vi "OpenMV_SelectLab.vi"(2 "ROI":T1, 3 "image":picture) -> (0 "ROI out":T1, 1 "thresholds":dbl[](array[numeric])=[90.0, 10.0, 20.0, -20.0, 20.0, -20.0])   [LabVIEW 2017]
doc: "This VI pops up a window where the user can select a region of interest."
panel:
  out "Plots":T2
  out "Mouse Down":cluster{"X":i32, "Y":i32}
  out "String":string
  out "Mouse in":bool
  in  "Pen":u32(colorbox)=16774656
  out "overlay":picture caption="Image"
  in  "OK":bool
  out "Display":picture caption="new picture"
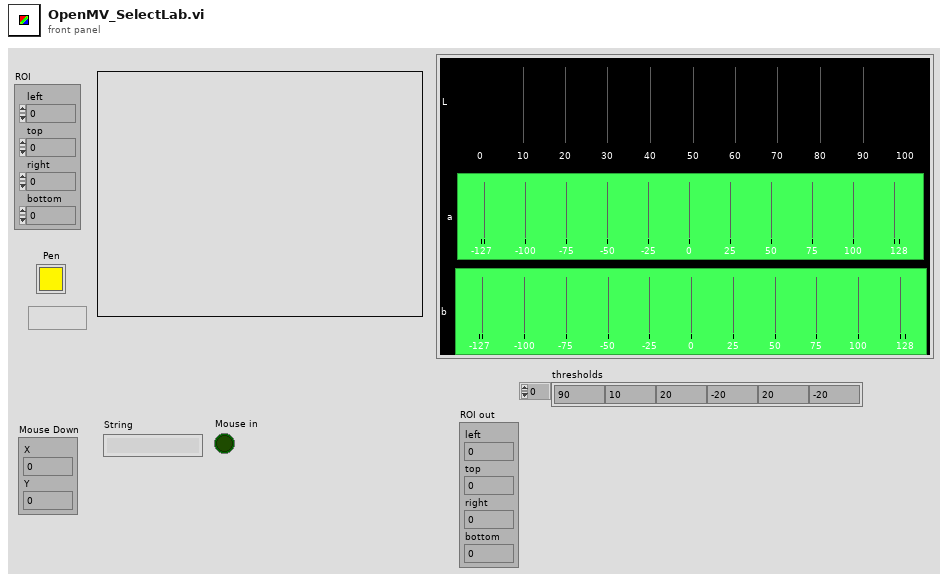
[diagram p1: front panel]
types:
  T1 = cluster{"left":i32, "top":i32, "right":i32, "bottom":i32}
  T2 = cluster{"L":dbl[], "a":cluster{i32, i32, dbl[]}, "b":cluster{i32, i32, dbl[]}}
  T3 = typedef "imagedata.ctl" = cluster{"image type":i32, "image depth":i32, "image":u8[], "mask":u8[], "colors":u32[], "Rectangle":cluster{"left":i16, "top":i16, "right":i16, "bottom":i16}}
  T4 = typedef "LVMouseTypeDef.ctl" = cluster{"Mouse Position":cluster{"X":i32, "Y":i32}, "Mouse Modifiers":cluster{"Button Down":bool, "Shift Mod":bool, "Menu Mod":bool, "Option Mod":bool}}
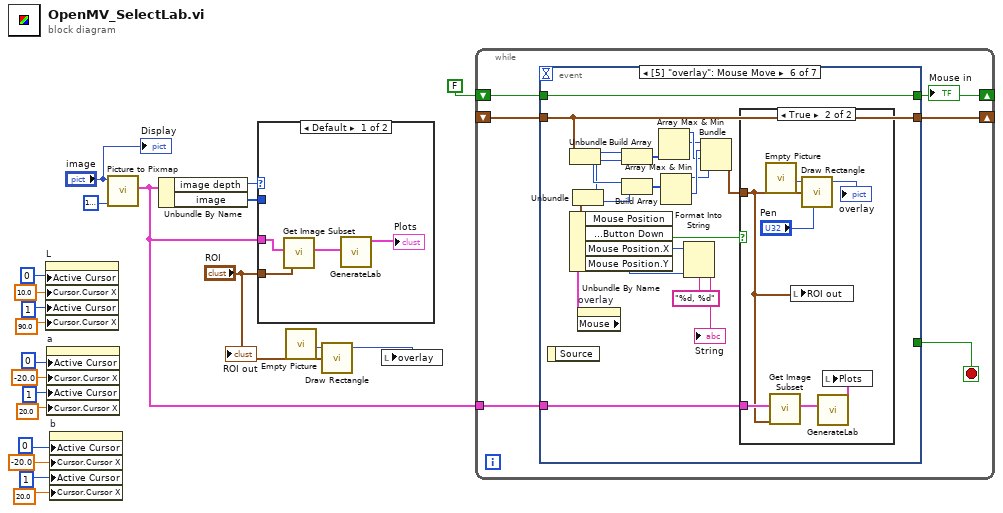
[diagram p0: block diagram]
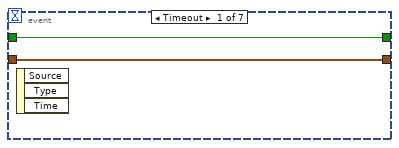
[diagram p3: hidden frame]
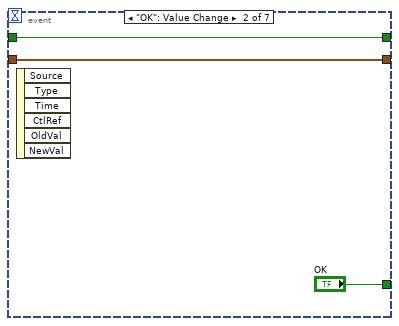
[diagram p4: hidden frame]
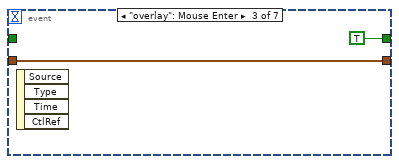
[diagram p5: hidden frame]
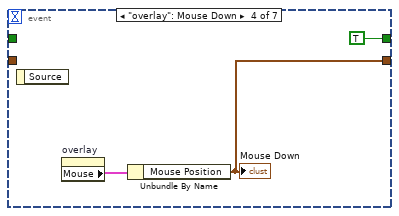
[diagram p6: hidden frame]
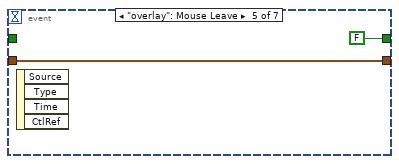
[diagram p7: hidden frame]
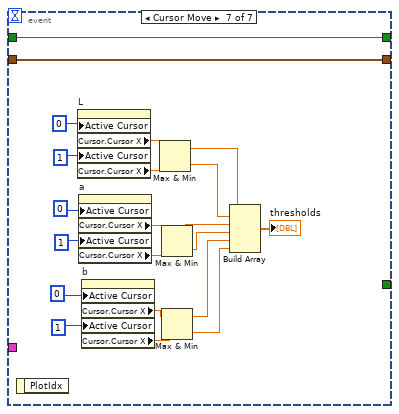
[diagram p9: hidden frame]
diagram:
  n1 = property on="L" class="WFGraph (strict)"("Active Cursor"=u32 0, "Cursor.Cursor X"=10.0 ("Cursor.Cursor Position:Cursor X"), "Active Cursor"=u32 1, "Cursor.Cursor X"=90.0 ("Cursor.Cursor Position:Cursor X")) -> ()  [unwired: 2 in, 2 out]
  n2 = property on="a" class="WFGraph (strict)"("Active Cursor"=u32 0, "Cursor.Cursor X"=-20.0 ("Cursor.Cursor Position:Cursor X"), "Active Cursor"=u32 1, "Cursor.Cursor X"=20.0 ("Cursor.Cursor Position:Cursor X")) -> ()  [unwired: 2 in, 2 out]
  n3 = property on="b" class="WFGraph (strict)"("Active Cursor"=u32 0, "Cursor.Cursor X"=-20.0 ("Cursor.Cursor Position:Cursor X"), "Active Cursor"=u32 1, "Cursor.Cursor X"=20.0 ("Cursor.Cursor Position:Cursor X")) -> ()  [unwired: 2 in, 2 out]
  n4 = call <vilib>:"Picture to Pixmap.vi"("Background Color"=u32 16777216, "picture"="image") -> ("image data"=w16:T3)  [unwired: 8 in, 1 out]
  n5 = Unbundle By Name(w16) -> ("image depth"=w19:i32, "image"=w18:u8[])
  n6 = case shown="Default" w19 {
    tunnel: w18 -> [_ _]
    tunnel: w16 -> [w24 _]
    tunnel: "ROI" -> [w22 _]
    frame Default {
      n7 = call <vilib>:"Get Image Subset.vi"("subset rect"=w22, "image data"=w24) -> ("image subset"=w23:T3)  [unwired: 4 in, 1 out]
      n8 = call "GenerateLab.vi"("image data"=w23) -> ("Plots"=→"Plots":T2)  [unwired: 9 in, 1 out]
    }
    frame ..8 {
    }
  }
  n9 = call "Empty Picture"() -> ("empty picture"=w3:picture)
  n10 = call <vilib>:"Draw Rectangle.vi"("picture"=w3, "rect"="ROI") -> ("new picture"=w1:picture)  [unwired: 7 in]
  n11 = local write "overlay"(w1) -> ()
  n12 = while {
    shift-right: [w30] -> _
    shift-left: FALSE ("Mouse in") -> [w29]
    shift-right: [w28] -> _
    shift-left: _ -> [w27]
    tunnel: w16 -> [w26]
    stop <- w31 stop-if-true
    n13 = event shown="[5] \"overlay\": Mouse Move" {
      selector: _ -> [_ _ _ _ _ _ _]
      dyn-events: _ -> [_ _ _ _ _ _ _]
      timeout: _ -> [_ _ _ _ _ _ _]
      tunnel: [_ "OK" _ _ _ _ _] -> w31
      tunnel: [w33 w35 TRUE ("Mouse in") TRUE ("Mouse in") FALSE ("Mouse in") w64 w91] -> w30
      tunnel: w29 -> [w33 w35 _ _ _ w64 w91]
      tunnel: [w32 w34 w37 w39 w42 w52 w92] -> w28
      tunnel: w27 -> [w32 w34 w37 _ w42 w52 w92]
      tunnel: w26 -> [_ _ _ _ _ w44 _]
      event Timeout {
        n14 = event-data() -> ()  [unwired: 1 in, 3 out]
      }
      event "OK": Value Change {
        n15 = event-data() -> ()  [unwired: 1 in, 6 out]
      }
      event "overlay": Mouse Enter {
        n16 = event-data() -> ()  [unwired: 1 in, 4 out]
      }
      event "overlay": Mouse Down {
        n17 = event-data() -> ()  [unwired: 1 in, 1 out]
        n18 = property on="overlay" class="Pict"() -> ("Mouse"=w40:T4)  [unwired: 2 in, 2 out]
        n19 = Unbundle By Name(w40) -> ("Mouse Position"=w39:cluster{"X":i32, "Y":i32})
        "Mouse Down" <- w39
      }
      event "overlay": Mouse Leave {
        n20 = event-data() -> ()  [unwired: 1 in, 4 out]
      }
      event "overlay": Mouse Move {
        n21 = event-data() -> ()  [unwired: 1 in, 1 out]
        n22 = Unbundle(w52) -> ("X"=w53:i32, "Y"=w51:i32)
        n23 = property on="overlay" class="Pict"() -> ("Mouse"=w63:T4)  [unwired: 2 in, 2 out]
        n24 = Unbundle By Name(w63) -> ("Mouse Position"=w48:cluster{"X":i32, "Y":i32}, "Mouse Modifiers.Button Down"=w62:bool, "Mouse Position.X"=w60:i32, "Mouse Position.Y"=w59:i32)
        n25 = Unbundle(w48) -> ("X"=w47:i32, "Y"=w46:i32)
        n26 = Build Array(w53, w47) -> (w50:i32[])
        n27 = Build Array(w51, w46) -> (w49:i32[])
        n28 = Array Max & Min(array=w50) -> (max value=w55:i32, min value=w54:i32)  [unwired: 2 out]
        n29 = Array Max & Min(array=w49) -> (max value=w56:i32, min value=w57:i32)  [unwired: 2 out]
        n30 = Format Into String(format string="%d, %d", w60, w59) -> (resulting string=→"String":string)  [unwired: 2 in, 1 out]
        n31 = Bundle(w54, w57, w55, w56) -> (w45:cluster{i32, i32, i32, i32})  [unwired: 1 out]
        n32 = case shown="True" w62 {
          tunnel: w45 -> [_ w65]
          tunnel: w44 -> [_ w68]
          frame False {
          }
          frame True {
            n33 = call "Empty Picture"() -> ("empty picture"=w71:picture)
            n34 = call <vilib>:"Get Image Subset.vi"("subset rect"=w65, "image data"=w68) -> ("image subset"=w67:T3)  [unwired: 4 in, 1 out]
            n35 = local write "ROI out"(w65) -> ()
            n36 = call <vilib>:"Draw Rectangle.vi"("picture"=w71, "rect"=w65, "color(black)"="Pen") -> ("new picture"=→"overlay":picture)  [unwired: 6 in]
            n37 = call "GenerateLab.vi"("image data"=w67) -> ("Plots"=w66:T2)  [unwired: 9 in, 1 out]
            n38 = local write "Plots"(w66) -> ()
          }
        }
      }
      event "Plots.L", "Plots.a", "Plots.b": Cursor Move {
        n39 = event-data() -> ()  [unwired: 1 in, 1 out]
        n40 = property on="L" class="WFGraph (strict)"("Active Cursor"=u32 0, "Active Cursor"=u32 1) -> ("Cursor.Cursor X"=w82:dbl, "Cursor.Cursor X"=w83:dbl)  [unwired: 2 in, 2 out]
        n41 = property on="a" class="WFGraph (strict)"("Active Cursor"=u32 0, "Active Cursor"=u32 1) -> ("Cursor.Cursor X"=w79:dbl, "Cursor.Cursor X"=w78:dbl)  [unwired: 2 in, 2 out]
        n42 = property on="b" class="WFGraph (strict)"("Active Cursor"=u32 0, "Active Cursor"=u32 1) -> ("Cursor.Cursor X"=w75:dbl, "Cursor.Cursor X"=w74:dbl)  [unwired: 2 in, 2 out]
        n43 = Max & Min(x=w82, y=w83) -> (max(x,y)=w81:dbl, min(x,y)=w80:dbl)
        n44 = Max & Min(x=w79, y=w78) -> (max(x,y)=w77:dbl, min(x,y)=w76:dbl)
        n45 = Max & Min(x=w75, y=w74) -> (max(x,y)=w73:dbl, min(x,y)=w72:dbl)
        n46 = Build Array(w81, w80, w77, w76, w73, w72) -> (→"thresholds":dbl[])
      }
    }
    "Mouse in" <- w30
  }
  "Display" <- "image"
  "ROI out" <- "ROI"
